vi "Send_Billede.vi"() -> ()   [LabVIEW 2018]
uses:
  <vilib>/myRIO/Instrument Drivers/Onboard IO/UART/typedef/VISA Configuration.ctl
  <vilib>/Instr/_visa.llb/VISA Configure Serial Port (Instr).vi
  <vilib>/myRIO/Express VI/Onboard IO/UART/UART Express VI.xnode
  <vilib>/myRIO/Instrument Drivers/Onboard IO/UART/UART.lvlib
panel:
  out "length of SH string":i32
  out "spreadsheet string":string
  out "Length of row":i32
  out "Picture from local variable":u8[][](graph)
  out "Picture that is send":u8[][](graph)
  out "Subarray send.":u8[](array[numeric])
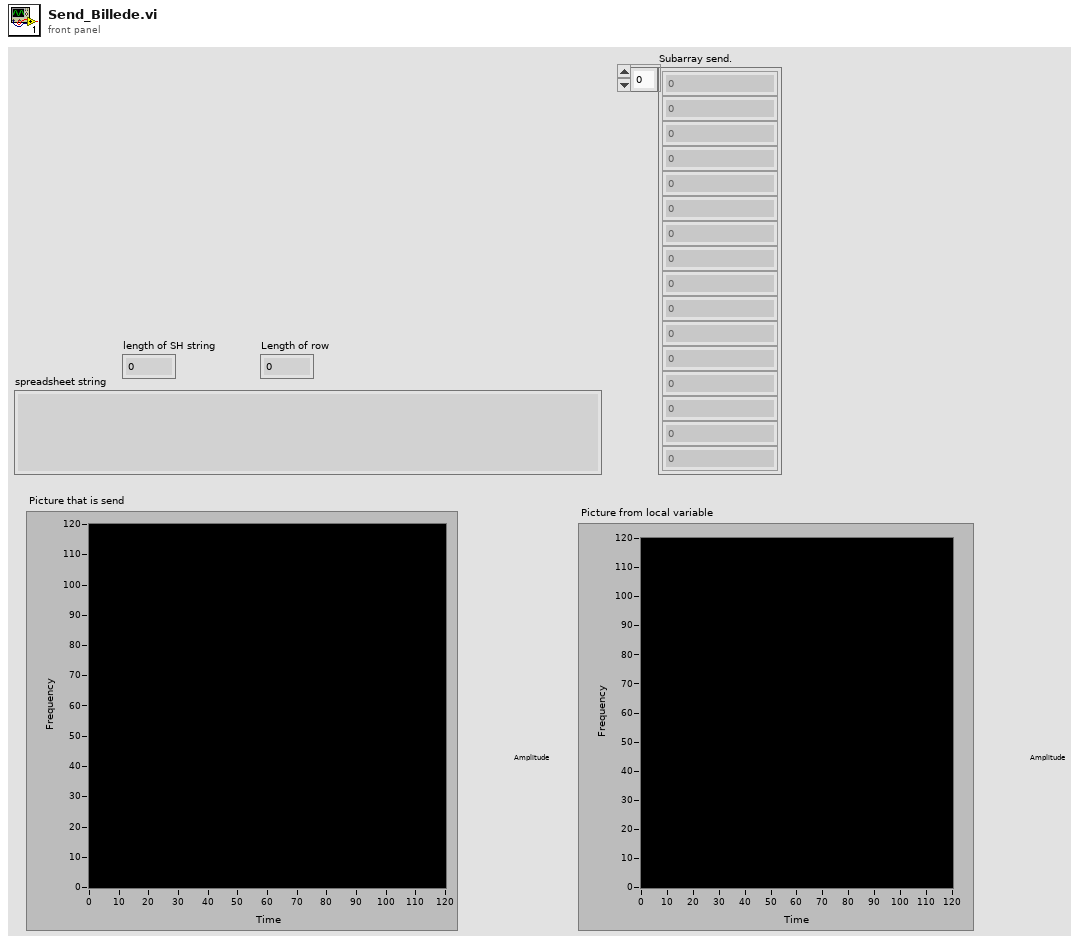
[diagram p1: front panel]
types:
  T1 = typedef "UART.lvlib/VISA Configuration.ctl" = cluster{"baud rate (9600)":u32, "data bits (8)":u16, "parity (0:none)":enum16{"None", "Odd", "Even", "Mark", "Space"}, "stop bits (10: 1 bit)":u16, "flow control (0:none)":u16, "termination char\n(0xA = '\\n' = LF) ":u8, "Enable Termination\nChar (T)":bool, "timeout (10sec)":u32}
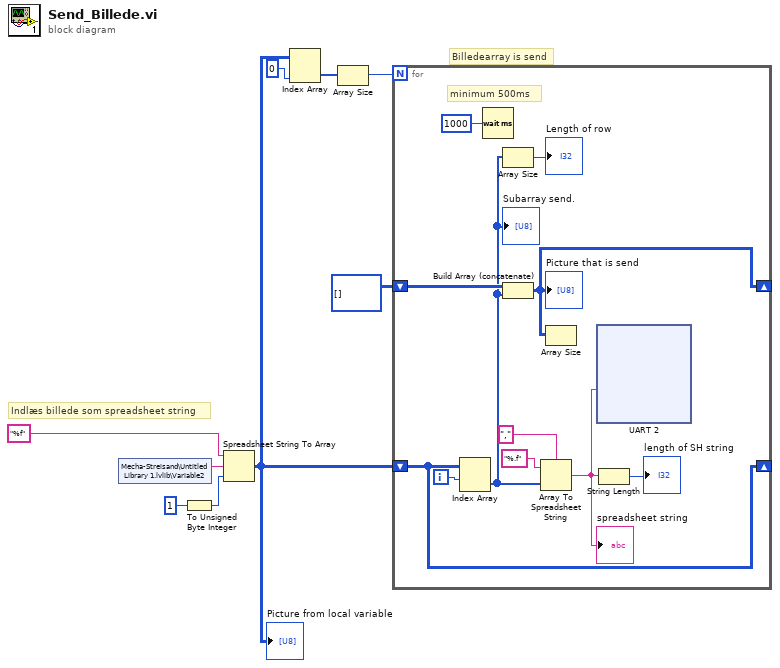
[diagram p0: block diagram]
diagram:
  # "Indlæs billede som spreadsheet string"
  # "Billedearray is send"
  n1 = shared-variable "Mecha-Streisand\\Untitled Library 1.lvlib\\Variable2"() -> (w8:string)  [unwired: 1 in, 1 out]
  n2 = To Unsigned Byte Integer(number=u8 1) -> (unsigned 8bit integer=w7:u8)
  n3 = Spreadsheet String To Array(format string="%f", spreadsheet string=w8, array type (2D Dbl)=w7) -> (array=w4:u8[][])  [unwired: 1 in]
  "Picture from local variable" <- w4
  n4 = Index Array(array=w4, index (col)=0 ("disabled index (col)")) -> (element=w2:u8[])  [unwired: 1 in]
  n5 = Array Size(array=w2) -> (size(s)=w1:i32)
  n6 = for {
    N: w1 -> [_]
    shift-right: [w20] -> _
    shift-left: w4 -> [w20]
    shift-right: [w14] -> _
    shift-left: u8[][] [] -> [w19]
    i -> [w18]
    # "minimum 500ms"
    n7 = Index Array(array=w20, index (row)=w18) -> (element=w12:u8[])  [unwired: 1 in]
    "Subarray send." <- w12
    n8 = Wait (ms)(milliseconds to wait=u32 1000) -> ()  [unwired: 1 out]
    n9 = Array Size(array=w12) -> (size(s)=→"Length of row":i32)
    n10 = Build Array (concatenate)(w19, w12) -> (w14:u8[][])
    "Picture that is send" <- w14
    n11 = Array To Spreadsheet String(delimiter (Tab)=",", array=w12, 3:"%.f" ("format string")) -> (spreadsheet string=w11:string)
    "spreadsheet string" <- w11
    n12 = Array Size(array=w14) -> ()  [unwired: 1 out]
    n13 = xnode "UART 2"("Characters to Write"=w11) -> ()  [unwired: 1 in, 2 out]
    n14 = String Length(string=w11) -> (length=→"length of SH string":i32)
  }
